vi "Measure Output.vi"(8 "error in (no error)":errorcluster, 11 "IF_XX in":refnum<class "IF_XX.lvclass">) -> (0 "error out":errorcluster, 1 "Current":dbl[](array[numeric]), 2 "Voltage":dbl[](array[numeric]), 3 "IF_XX out":refnum<class "IF_XX.lvclass">)   [LabVIEW 2019, in "IF_XX.lvlib" / "IF_XX.lvclass"]
doc: "This VI is the device specific query of current and voltage measurements. \nThe return values are: \nVoltage Array - One voltage measurement per channel single channel supplies should only return a single array element\nCurrent Array - - One current measurement per channel single channel supplies should only return a single array element\n\n***NOTE***\nThis override calls the commercial library to perform the operation. The VI's reentrancy settings are indeterminate, and therefore there is a risk for functional contention causing increasing cascading delays if multiple power supplies are used."
uses:
  Library/IF_XX.lvclass
  Library/IF_XX.lvclass/IF_XX.ctl
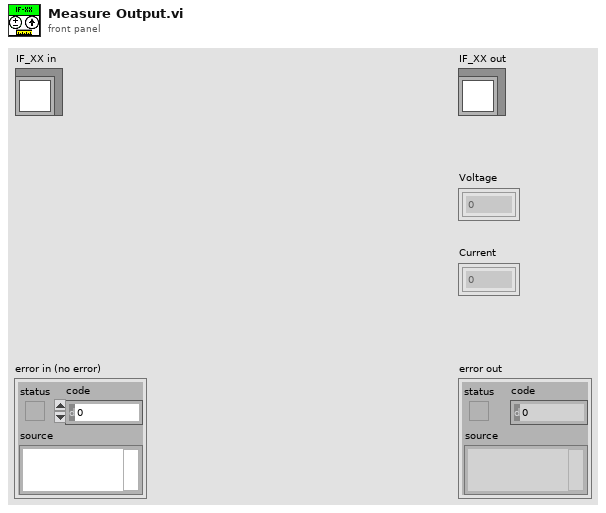
[diagram p1: front panel]
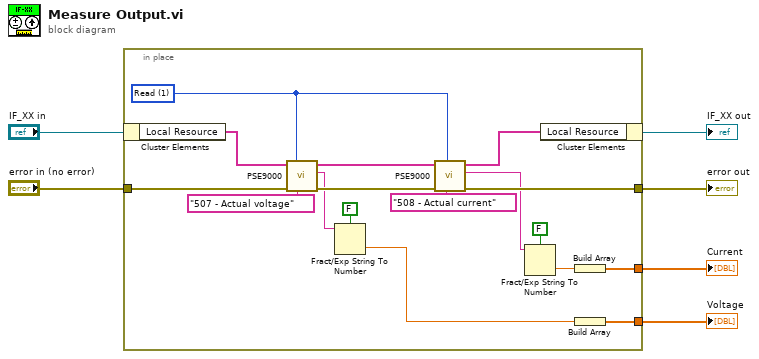
[diagram p0: block diagram]
diagram:
  n1 = in-place {
    in-place-border: "error in (no error)" -> [w17]
    in-place-border: [w16] -> w4
    in-place-border: [w8] -> w2
    in-place-border: [w7] -> w1
    w20 = u8 1 items=["Write", "Read"] ("Access")
    n2 = in-place-cluster #1("IF_XX in") -> ("Local Resource"=w22:string[])
    n3 = call <instrlib>:"PSE9000.vi"("Command list"="507 - Actual voltage", "Error in"=w17, "Access"=w20, "Device information in"=w22) -> ("Error out"=w18:errorcluster, "Read data"=w14:string, "Device information out"=w23:string[])  [unwired: 2 in, 1 out]
    n4 = Fract/Exp String To Number(use system decimal point (T)=FALSE, string=w14) -> (number=w9:dbl)  [unwired: 2 in, 1 out]
    n5 = call <instrlib>:"PSE9000.vi"("Command list"="508 - Actual current", "Error in"=w18, "Access"=w20, "Device information in"=w23) -> ("Error out"=w16:errorcluster, "Read data"=w13:string, "Device information out"=w21:string[])  [unwired: 2 in, 1 out]
    n6 = Fract/Exp String To Number(use system decimal point (T)=FALSE, string=w13) -> (number=w10:dbl)  [unwired: 2 in, 1 out]
    n7 = in-place-cluster #1("Local Resource"=w21) -> (→"IF_XX out":refnum<class "IF_XX.lvclass">)
    n8 = Build Array(w10) -> (w8:dbl[])
    n9 = Build Array(w9) -> (w7:dbl[])
  }
  "error out" <- w4
  "Current" <- w2
  "Voltage" <- w1
